vi "Manual Assembly DB_12_4_2024.vi"() -> ()   [LabVIEW 2021]
uses:
  Classes/Routine/Routine Enum.ctl
  Classes/Assembly/Database Entry/Database Entry.lvclass
  Classes/Assembly/Assembly Run.lvclass
  Classes/Workspace/Fixture Enum.ctl
  <vilib>/Utility/file.llb/Read Delimited Spreadsheet (string).vi
  SubVIs/PUT_region.vi
  SubVIs/component_tray_region.vi
  SubVIs/assembly_tray_region.vi
  Classes/Routine/Routine.lvclass
  Classes/Workspace/Fixture.lvclass
  Classes/Controller/Controller.lvclass
  <vilib>/JDP Science/JDP Science Common Utilities/JDP Utility.lvlib
panel:
  out "Stack names":T1
  out "Feet check":bool
  out "Assembly Type":string[](array[string])
  out "Assembly tray region":dbl
  out "Component tray region":dbl
  out "PUT Region":dbl
  in  "Clear All":bool
  in  "Assemble":bool
  in  "Pick and Place":bool
  in  "Dispense glue":bool
  in  "Go":bool
  in  "Routine":T2=enum."Dispense Epoxy"
  in  "Update":bool
  in  "Stage":i32(listbox)=-1
  in  "Stop":bool
  in  "Remove":bool
  in  "Add":bool
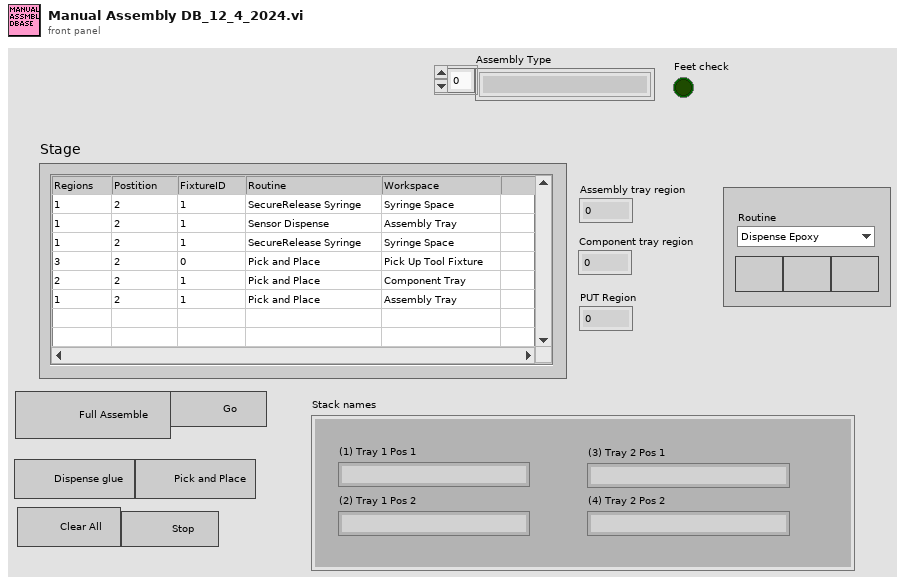
[diagram p1: front panel]
types:
  T1 = cluster{"(1) Tray 1 Pos 1":string, "(2) Tray 1 Pos 2":string, "(3) Tray 2 Pos 1":string, "(4) Tray 2 Pos 2":string}
  T2 = typedef "Routine.lvclass/Routine Enum.ctl" = enum16{"Primary Pick Up", "Secondary Pick Up", "Put Down All", "Secure Syringe", "Release Syringe", "Dispense Epoxy", "Pick Up All", "Put Down Secondary", "Full Assembly"}
  T3 = typedef "Fixture.lvclass/Fixture Enum.ctl" = enum16{"Assembly Tray", "Syringe Space", "Component", "Pick Up Tool", "Current Position"}
  T4 = typedef "File Paths.ctl" = cluster{"Glue Pattern Folder":path, "Carrier Tray Folder":path, "Pick Up Tool Fixture Folder":path, "Components Folder":path, "Bellows Tool Offset.txt":path, "Pick Up Tool Offset.txt":path, "Dispense Tip Offset.txt":path, "Log Files":path, "Gantry Assembly Map.txt":path, "Syringe and offset map.txt":path, "Controllers Folder":path, "Local dbase config":path}
  T5 = cluster{"Fixture ID":dbl, "Position":dbl, "Thickness":dbl}[]
  T6 = cluster{"Stack names[0]":string, "Stack names[1]":string, "Stack names[2]":string, "Stack names[3]":string}
  T7 = typedef "Controller.lvclass/Controllers.ctl" = cluster{"I-O.lvclass":refnum<class "I-O.lvclass">, "Gantry":refnum<k24>, "Dispenser":refnum<visa-resource-name>}
  T8 = cluster{"Fixture ID":dbl, "Position":dbl, "Thickness":dbl}
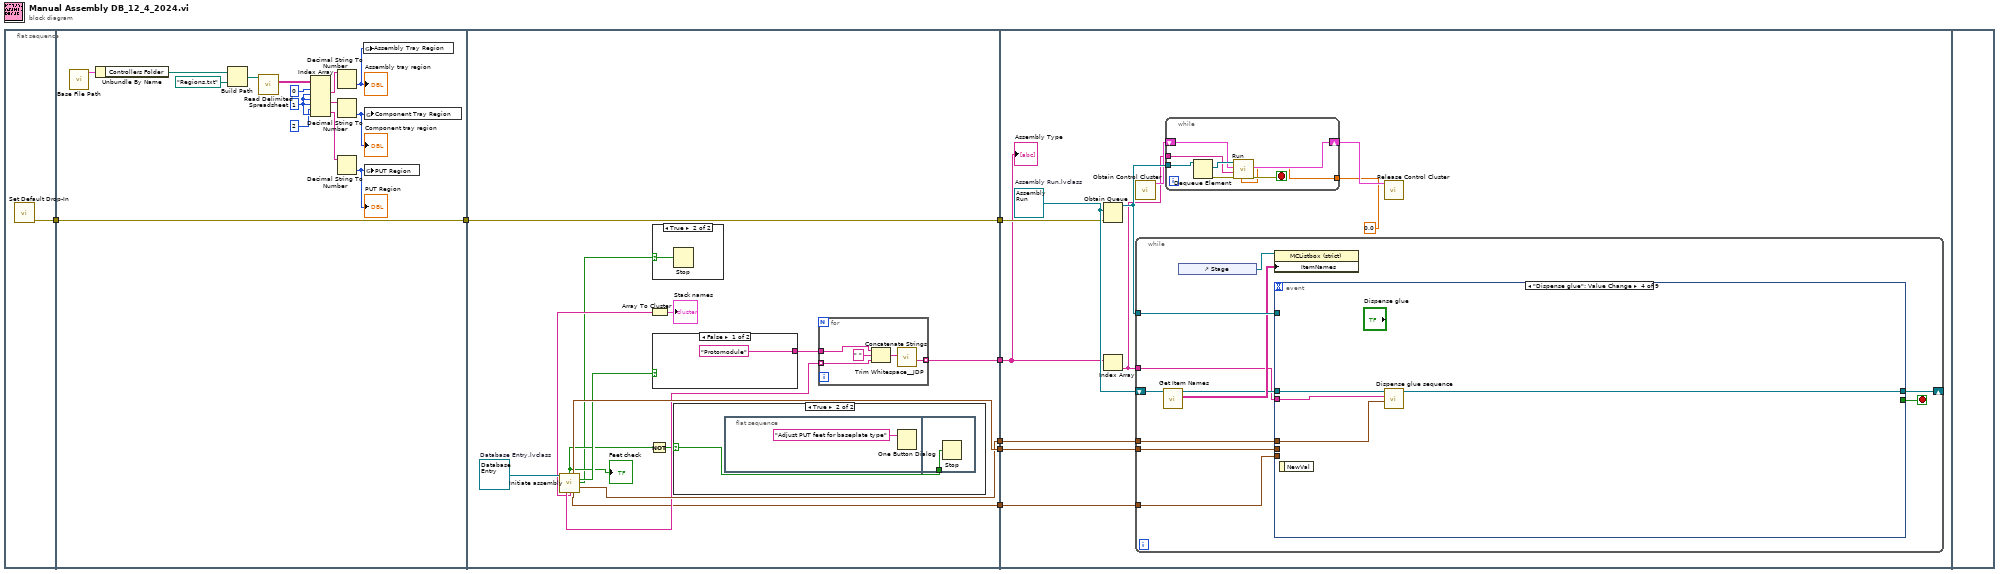
[diagram p0: block diagram]
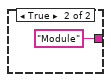
[diagram p4: hidden frame]
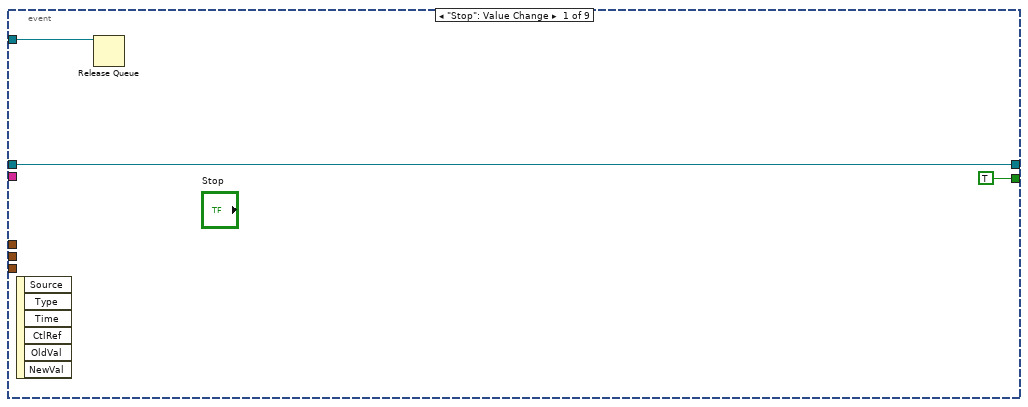
[diagram p5: hidden frame]
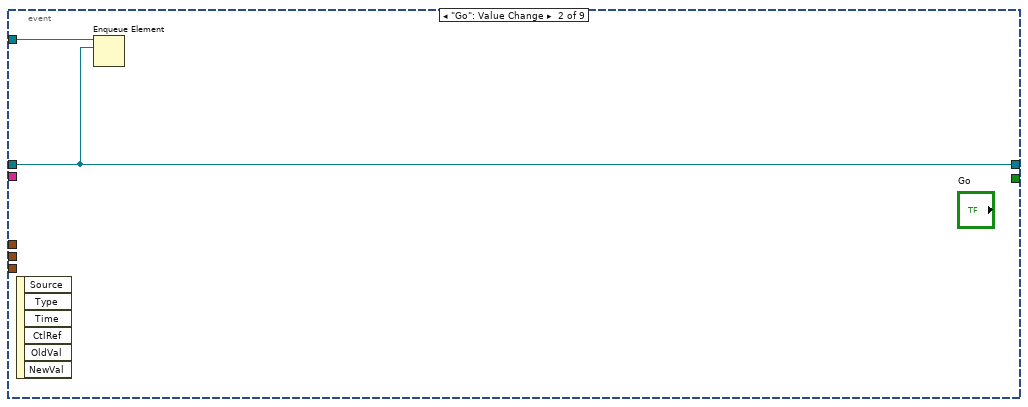
[diagram p6: hidden frame]
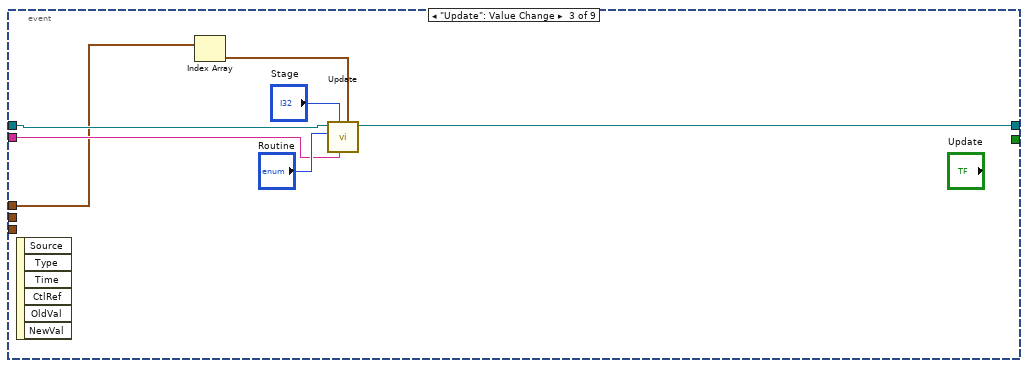
[diagram p7: hidden frame]
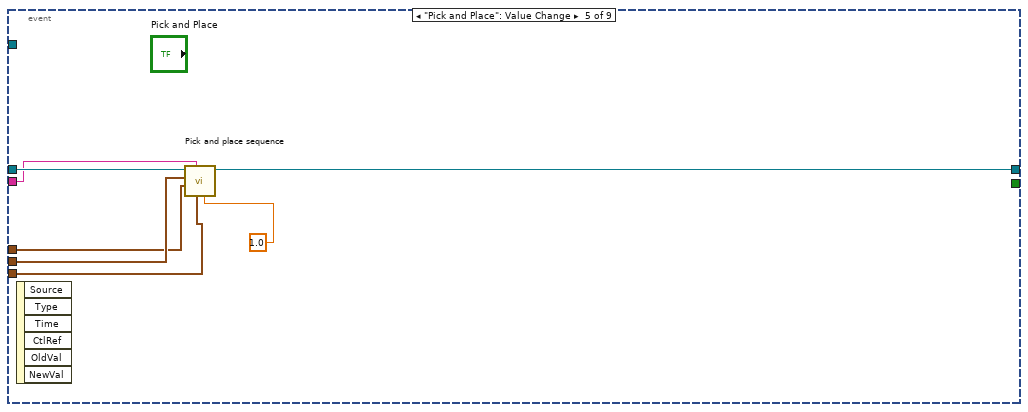
[diagram p8: hidden frame]
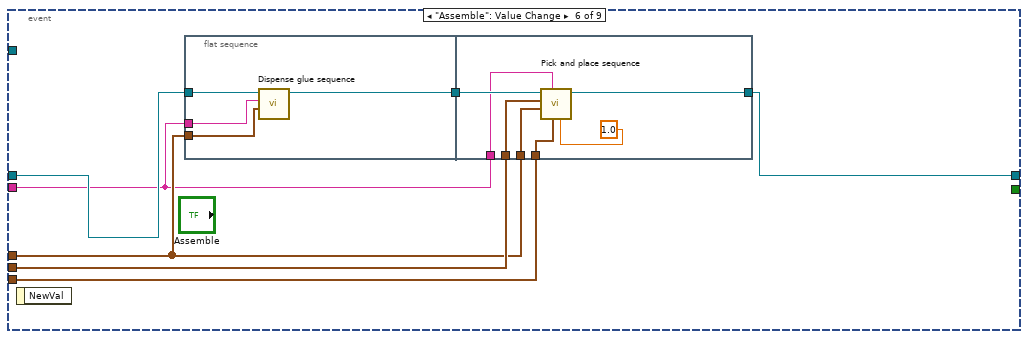
[diagram p9: hidden frame]
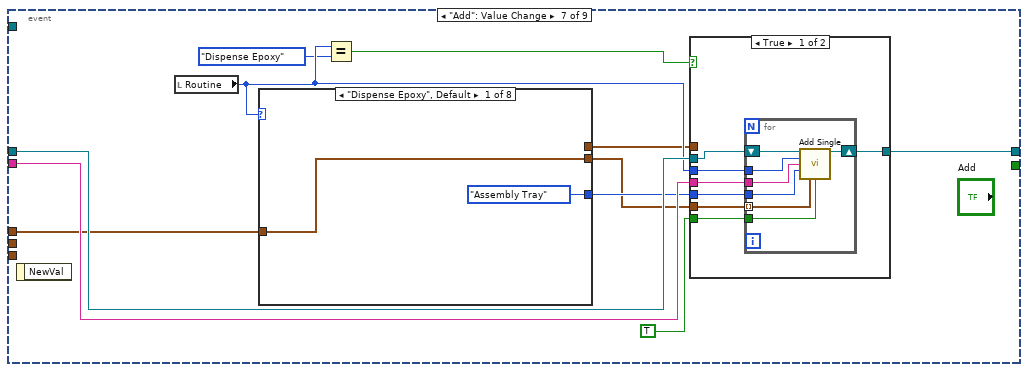
[diagram p10: hidden frame]
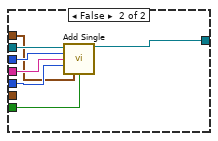
[diagram p11: hidden frame]
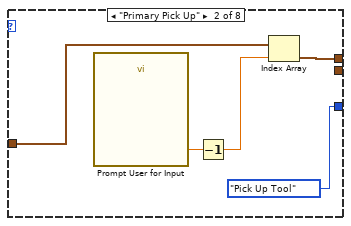
[diagram p12: hidden frame]
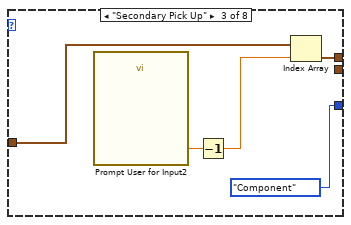
[diagram p13: hidden frame]
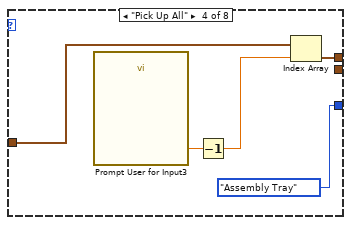
[diagram p14: hidden frame]
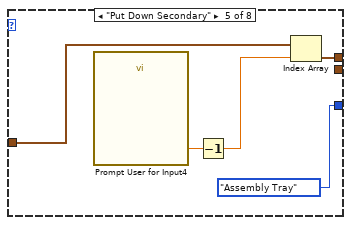
[diagram p15: hidden frame]
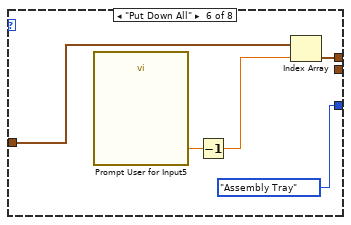
[diagram p16: hidden frame]
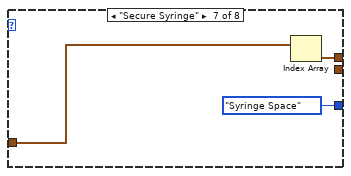
[diagram p17: hidden frame]
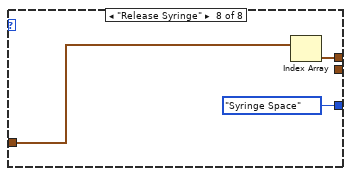
[diagram p18: hidden frame]
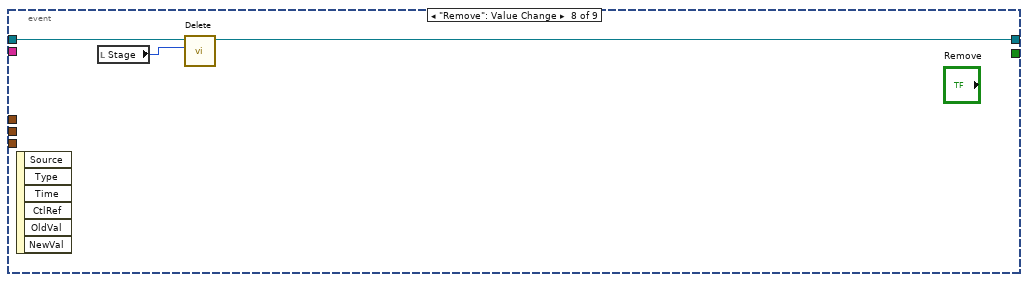
[diagram p19: hidden frame]
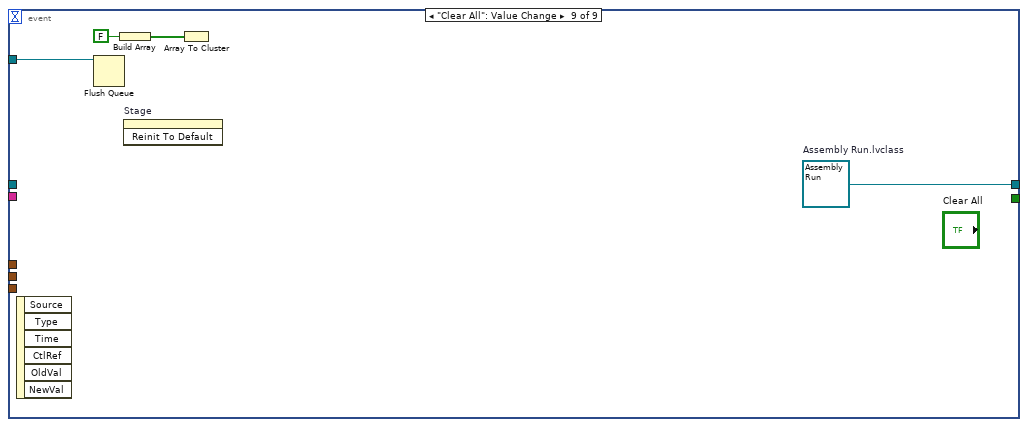
[diagram p20: hidden frame]
diagram:
  n1 = flat-sequence {
    tunnel: [w8] -> w5
    tunnel: [w9] -> w6
    tunnel: w5 -> [w9]
    tunnel: [w36] -> w7
    tunnel: w6 -> [w36]
    tunnel: [w24] -> w4
    tunnel: [w35] -> w3
    tunnel: [w34] -> w2
    tunnel: [w30] -> w1
    tunnel: w7 -> [w55]
    tunnel: w4 -> [w54]
    tunnel: w3 -> [w53]
    tunnel: w2 -> [w52]
    tunnel: w1 -> [w51]
    frame #0 {
      n2 = call "Set Default Drop-In.vi"() -> ("error out"=w8:errorcluster)  [unwired: 11 in]
    }
    frame #1 {
      w12 = 1 ("disabled index (col)")
      n3 = call "Base File Path.vi"() -> ("Paths Out"=w23:T4)  [unwired: 11 in]
      n4 = Unbundle By Name(w23) -> ("Controllers Folder"=w21:path)
      n5 = Build Path(base path=w21, name or relative path=path "Regions.txt") -> (appended path=w22:path)
      n6 = call-poly <vilib>:"Read Delimited Spreadsheet.vi"("file path (dialog if empty)"=w22) -> ("all rows"=w10:string[][])  [unwired: 9 in, 5 out]
      n7 = Index Array(array=w10, index (row) #1=0 ("index (row)"), index (col) #1=w12, index (row) #2=w12, index (col) #2=w12, index (row) #3=2 ("disabled index (row)"), index (col) #3=w12) -> (element #1=w15:string, element #2=w14:string, element #3=w16:string)
      n8 = Decimal String To Number(string=w15) -> (number=w18:i32)  [unwired: 2 in, 1 out]
      "Assembly tray region" <- w18
      n9 = Decimal String To Number(string=w14) -> (number=w19:i32)  [unwired: 2 in, 1 out]
      "Component tray region" <- w19
      n10 = Decimal String To Number(string=w16) -> (number=w17:i32)  [unwired: 2 in, 1 out]
      "PUT Region" <- w17
      n11 = global write "assembly_tray_region.vi" "Assembly Tray Region"(w18) -> ()
      n12 = global write "component_tray_region.vi" "Component Tray Region"(w19) -> ()
      n13 = global write "PUT_region.vi" "PUT Region"(w17) -> ()
    }
    frame #2 {
      w37 = refnum<class "Database Entry.lvclass"> refnum  # Database Entry.lvclass
      n14 = call "Initiate assembly.vi"("Database Entry in"=w37) -> ("Feet check"=w26:bool, "PUT Settings"=w35:T5, "Module?"=w33:bool, "Abort out"=w25:bool, "Assembly Settings"=w34:T5, "Assembly Type"=w32:string[], "Stack names"=w27:string[], "Component Settings"=w24:T5)  [unwired: 5 in, 2 out]
      "Feet check" <- w26
      n15 = Array To Cluster(array=w27) -> (cluster=→"Stack names":T6)
      n16 = Not(x=w26) -> (.not. x?=w29:bool)
      n17 = case shown="True" w25 {
        selector: w25 -> [_ w38]
        frame False {
        }
        frame True {
          n18 = Stop(stop? (T)=w38) -> ()
        }
      }
      n19 = case shown="False" w33 {
        tunnel: ["Protomodule" "Module"] -> w31
        frame False {
        }
        frame True {
        }
      }
      n20 = case shown="True" w29 {
        selector: w29 -> [_ w39]
        frame False {
        }
        frame True {
          n21 = flat-sequence {
            tunnel: w39 -> [w41]
            frame #0 {
              n22 = One Button Dialog(message="Adjust PUT feet for baseplate type") -> ()  [unwired: 1 in, 1 out]
            }
            frame #1 {
              n23 = Stop(stop? (T)=w41) -> ()
            }
          }
        }
      }
      n24 = for {
        tunnel: w32 -> [w44] mode=indexing
        tunnel: w31 -> [w46]
        tunnel: [w42] -> w30 mode=indexing
        n25 = Concatenate Strings(w46, " " ("string"), w44) -> (w43:string)
        n26 = call <vilib>:"Trim Whitespace__JDP.vi"("String in"=w43) -> ("String out"=w42:string)  [unwired: 6 in]
      }
    }
    frame #3 {
      w57 = refnum<class "Assembly Run.lvclass"> refnum  # Assembly Run.lvclass
      n27 = Obtain Queue(element data type=w57, error in (no error)=w55) -> (queue out=w59:refnum<queue>)  [unwired: 3 in, 2 out]
      n28 = Index Array(array=w51) -> (element=w50:string)  [unwired: 1 in]
      n29 = call "Obtain Control Cluster.vi"() -> ("Control Out"=w56:T7)  [unwired: 11 in]
      n30 = while {
        shift-right: [w64] -> _
        shift-left: w57 -> [w66]
        tunnel: w59 -> [w69]
        tunnel: w54 -> [w63]
        tunnel: w53 -> [w62]
        tunnel: w52 -> [w61]
        tunnel: w50 -> [w60]
        stop <- w70 stop-if-true
        n31 = call "Get Item Names.vi"("Assembly Run in"=w66) -> ("Item names"=w68:string[][], "Assembly Run out"=w65:refnum<class "Assembly Run.lvclass">)  [unwired: 8 in, 1 out]
        n32 = control-ref of="Stage"() -> (w67:refnum<vi>)
        n33 = property class="MCListbox (strict)"(reference=w67, "ItemNames"=w68) -> ()  [unwired: 1 in, 2 out]
        n34 = event shown="[3] \"Dispense glue\": Value Change" {
          selector: _ -> [_ _ _ _ _ _ _ _ _]
          dyn-events: _ -> [_ _ _ _ _ _ _ _ _]
          timeout: _ -> [_ _ _ _ _ _ _ _ _]
          tunnel: [TRUE _ _ _ _ _ _ _ _] -> w70
          tunnel: w65 -> [w72 w74 w82 w86 w93 w100 w121 w179 _]
          tunnel: [w72 w74 w81 w85 w92 w99 w122 w178 w183] -> w64
          tunnel: w69 -> [w71 w75 _ _ _ _ _ _ w182]
          tunnel: w63 -> [_ _ _ _ w88 w96 _ _ _]
          tunnel: w62 -> [_ _ _ _ w91 w97 _ _ _]
          tunnel: w61 -> [_ _ w77 w84 w87 w95 w117 _ _]
          tunnel: w60 -> [_ _ w78 w83 w90 w94 w120 _ _]
          event "Stop": Value Change {
            n35 = event-data() -> ()  [unwired: 1 in, 6 out]
            n36 = Release Queue(queue=w71) -> ()  [unwired: 2 in, 3 out]
          }
          event "Go": Value Change {
            n37 = event-data() -> ()  [unwired: 1 in, 6 out]
            n38 = Enqueue Element(queue=w75, element=w74) -> ()  [unwired: 2 in, 3 out]
          }
          event "Update": Value Change {
            n39 = event-data() -> ()  [unwired: 1 in, 6 out]
            n40 = Index Array(array=w77) -> (element=w76:T8)  [unwired: 1 in]
            n41 = call "Update.vi"("Input Settings"=w76, "Assembly Type"=w78, "Row"="Stage", "Routine"="Routine", "Assembly Run in"=w82) -> ("Assembly Run out"=w81:refnum<class "Assembly Run.lvclass">)  [unwired: 5 in, 1 out]
          }
          event "Dispense glue": Value Change {
            n42 = event-data() -> ()  [unwired: 1 in, 1 out]
            n43 = call "Dispense glue sequence.vi"("Assembly Tray Settings Array"=w84, "Assembly Type"=w83, "Assembly Run in"=w86) -> ("Assembly Run out"=w85:refnum<class "Assembly Run.lvclass">)  [unwired: 7 in, 1 out]
          }
          event "Pick and Place": Value Change {
            n44 = event-data() -> ()  [unwired: 1 in, 6 out]
            n45 = call "Pick and place sequence.vi"("Numeric"=1.0, "Component Tray map"=w88, "Assembly Type"=w90, "Assembly Tray map"=w87, "PUT map"=w91, "Assembly Run in"=w93) -> ("Assembly Run out"=w92:refnum<class "Assembly Run.lvclass">)  [unwired: 4 in, 1 out]
          }
          event "Assemble": Value Change {
            n46 = event-data() -> ()  [unwired: 1 in, 1 out]
            n47 = flat-sequence {
              tunnel: [w103] -> w98
              tunnel: w100 -> [w104]
              tunnel: w95 -> [w102]
              tunnel: w94 -> [w101]
              tunnel: [w110] -> w99
              tunnel: w98 -> [w111]
              tunnel: w95 -> [w109]
              tunnel: w97 -> [w108]
              tunnel: w96 -> [w107]
              tunnel: w94 -> [w106]
              frame #0 {
                n48 = call "Dispense glue sequence.vi"("Assembly Tray Settings Array"=w102, "Assembly Type"=w101, "Assembly Run in"=w104) -> ("Assembly Run out"=w103:refnum<class "Assembly Run.lvclass">)  [unwired: 7 in, 1 out]
              }
              frame #1 {
                n49 = call "Pick and place sequence.vi"("Numeric"=1.0, "Component Tray map"=w107, "Assembly Type"=w106, "Assembly Tray map"=w109, "PUT map"=w108, "Assembly Run in"=w111) -> ("Assembly Run out"=w110:refnum<class "Assembly Run.lvclass">)  [unwired: 4 in, 1 out]
              }
            }
          }
          event "Add": Value Change {
            n50 = event-data() -> ()  [unwired: 1 in, 1 out]
            n51 = local read "Routine"() -> (w115:T2)
            n52 = case shown="\"Dispense Epoxy\", Default" w115 {
              tunnel: [Fixture_Enum."Assembly Tray" ("Fixture") Fixture_Enum."Pick Up Tool" ("Fixture") Fixture_Enum."Component" ("Fixture") Fixture_Enum."Assembly Tray" ("Fixture") Fixture_Enum."Assembly Tray" ("Fixture") Fixture_Enum."Assembly Tray" ("Fixture") Fixture_Enum."Syringe Space" ("Fixture") Fixture_Enum."Syringe Space" ("Fixture")] -> w119
              tunnel: w117 -> [w144 w149 w152 w157 w162 w166 w172 w175]
              tunnel: [_ w146 w151 w156 w161 w167 w171 w174] -> w112
              tunnel: [w144 _ _ _ _ _ _ _] -> w113
              frame "Dispense Epoxy", Default {
              }
              frame "Primary Pick Up" {
                n53 = call "Prompt User for Input"() -> ("Position"=w148:dbl)  [unwired: 17 in, 2 out]
                n54 = Decrement(x=w148) -> (x-1=w147:dbl)
                n55 = Index Array(array=w149, index=w147) -> (element=w146:T8)
              }
              frame "Secondary Pick Up" {
                n56 = call "Prompt User for Input2"() -> ("Position"=w154:dbl)  [unwired: 17 in, 2 out]
                n57 = Decrement(x=w154) -> (x-1=w153:dbl)
                n58 = Index Array(array=w152, index=w153) -> (element=w151:T8)
              }
              frame "Pick Up All" {
                n59 = call "Prompt User for Input3"() -> ("Position"=w159:dbl)  [unwired: 17 in, 2 out]
                n60 = Decrement(x=w159) -> (x-1=w158:dbl)
                n61 = Index Array(array=w157, index=w158) -> (element=w156:T8)
              }
              frame "Put Down Secondary" {
                n62 = call "Prompt User for Input4"() -> ("Position"=w164:dbl)  [unwired: 17 in, 2 out]
                n63 = Decrement(x=w164) -> (x-1=w163:dbl)
                n64 = Index Array(array=w162, index=w163) -> (element=w161:T8)
              }
              frame "Put Down All" {
                n65 = call "Prompt User for Input5"() -> ("Position"=w169:dbl)  [unwired: 17 in, 2 out]
                n66 = Decrement(x=w169) -> (x-1=w168:dbl)
                n67 = Index Array(array=w166, index=w168) -> (element=w167:T8)
              }
              frame "Secure Syringe" {
                n68 = Index Array(array=w172) -> (element=w171:T8)  [unwired: 1 in]
              }
              frame "Release Syringe" {
                n69 = Index Array(array=w175) -> (element=w174:T8)  [unwired: 1 in]
              }
            }
            n70 = Equal?(x=w115, y=Routine_Enum."Dispense Epoxy") -> (x = y?=w116:bool)
            n71 = case shown="True" w116 {
              tunnel: [w129 w143] -> w122
              tunnel: w121 -> [w128 w142]
              tunnel: w120 -> [w127 w141]
              tunnel: w119 -> [w126 w140]
              tunnel: w115 -> [w125 w139]
              tunnel: TRUE ("Auto") -> [w124 w138]
              tunnel: w113 -> [w123 _]
              tunnel: w112 -> [_ w137]
              frame True {
                n72 = for {
                  tunnel: w127 -> [w134]
                  tunnel: w126 -> [w133]
                  tunnel: w125 -> [w132]
                  tunnel: w124 -> [w131]
                  shift-right: [w136] -> w129
                  shift-left: w128 -> [w135]
                  tunnel: w123 -> [w130] mode=indexing
                  n73 = call-dynamic "Add Single.vi"("UI in"=w135, "Routine"=w132, "Assembly Type"=w134, "Fixture"=w133, "Input Settings"=w130, "Auto"=w131) -> ("UI out"=w136:refnum<class "Assembly Run.lvclass">)  [unwired: 8 in, 1 out]
                }
              }
              frame False {
                n74 = call-dynamic "Add Single.vi"("UI in"=w142, "Routine"=w139, "Assembly Type"=w141, "Fixture"=w140, "Input Settings"=w137, "Auto"=w138) -> ("UI out"=w143:refnum<class "Assembly Run.lvclass">)  [unwired: 8 in, 1 out]
              }
            }
          }
          event "Remove": Value Change {
            n75 = event-data() -> ()  [unwired: 1 in, 6 out]
            n76 = local read "Stage"() -> (w177:i32)
            n77 = call "Delete.vi"("Index"=w177, "Assembly In"=w179) -> ("Assembly Out"=w178:refnum<class "Assembly Run.lvclass">)  [unwired: 8 in, 1 out]
          }
          event "Clear All": Value Change {
            w183 = refnum<class "Assembly Run.lvclass"> refnum  # Assembly Run.lvclass
            n78 = event-data() -> ()  [unwired: 1 in, 6 out]
            n79 = Flush Queue(queue=w182) -> ()  [unwired: 1 in, 3 out]
            n80 = Build Array(FALSE) -> (w181:bool[])
            n81 = invoke on="Stage" class="MCListbox (strict)" method="Reinit To Default"() -> ()  [unwired: 3 in, 3 out]
            n82 = Array To Cluster(array=w181) -> ()  [unwired: 1 out]
          }
        }
      }
      n83 = while {
        tunnel: w59 -> [w191]
        shift-right: [w186] -> w58
        shift-left: w56 -> [w187]
        tunnel: w50 -> [w185]
        tunnel: 0.0 ("Pickup_Test_Number") -> [w184]
        stop <- w188 stop-if-true
        n84 = Dequeue Element(queue=w191) -> (element=w190:refnum<class "Assembly Run.lvclass">, error out=w189:errorcluster)  [unwired: 2 in, 2 out]
        n85 = call-dynamic "Run.vi"("Pickup_Test_Number"=w184, "error in (no error)"=w189, "Assembly Type"=w185, "Control In"=w187, "Assembly In"=w190) -> ("error out"=w188:errorcluster, "Control Out"=w186:T7)  [unwired: 4 in, 1 out]
      }
      n86 = call "Release Control Cluster.vi"("output cluster"=w58) -> ()  [unwired: 11 in]
      "Assembly Type" <- w51
    }
    frame #4 {
    }
  }
